vi "galvo_postns_fglobal.vi"(8 "error in (no error)":errorcluster, 9 "write?":bool, 10 "curr_y":dbl, 11 "curr_x":dbl) -> (0 "error out":errorcluster, 2 "curr_y":dbl, 3 "curr_x":dbl)   [LabVIEW 2015]
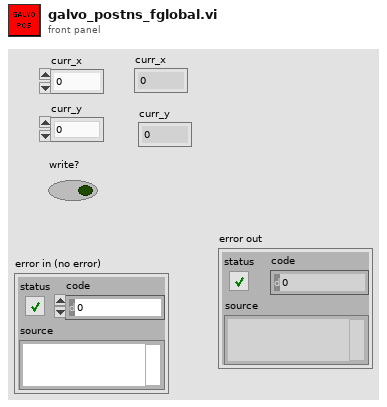
[diagram p1: front panel]
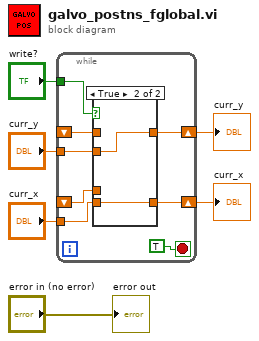
[diagram p0: block diagram]
diagram:
  n1 = while {
    shift-right: [w12] -> w2
    shift-left: _ -> [w11]
    tunnel: "curr_x" -> [w13]
    tunnel: "write?" -> [w14]
    shift-right: [w9] -> w3
    shift-left: _ -> [w10]
    tunnel: "curr_y" -> [w8]
    stop <- TRUE stop-if-true
    n2 = case shown="True" w14 {
      tunnel: w13 -> [_ w18]
      tunnel: [w16 w18] -> w12
      tunnel: w11 -> [w16 _]
      tunnel: w10 -> [w15 _]
      tunnel: [w15 w17] -> w9
      tunnel: w8 -> [_ w17]
      frame False {
      }
      frame True {
      }
    }
  }
  "curr_y" <- w3
  "curr_x" <- w2
  "error out" <- "error in (no error)"
